vi "Set Retardation in Wave Units.vi"(0 "VISA resource name":refnum<visa-resource-name>="COM1", 1 "fraction of wave":dbl min=0.0 max=1.0 step=0.001, 3 "error in (no error)":errorcluster) -> (7 "VISA resource name out":refnum<visa-resource-name>, 10 "error out":errorcluster)   [LabVIEW 2017]
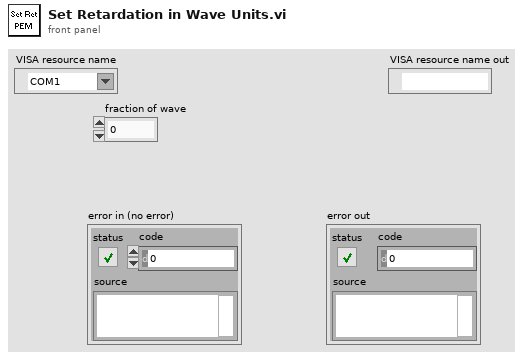
[diagram p1: front panel]
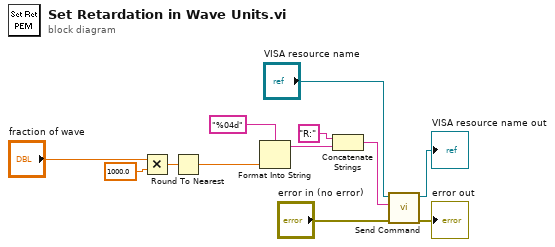
[diagram p0: block diagram]
diagram:
  n1 = Multiply(x="fraction of wave", y=1000.0) -> (x*y=w7:dbl)
  n2 = Round To Nearest(number=w7) -> (nearest integer value=w6:dbl)
  n3 = Format Into String(format string="%04d", w6) -> (resulting string=w10:string)  [unwired: 2 in, 1 out]
  n4 = Concatenate Strings("R:" ("write buffer"), w10) -> (w4:string)
  n5 = call "Send Command.vi"("error in (no error)"="error in (no error)", "write buffer"=w4, "VISA resource name"="VISA resource name") -> ("error out"=→"error out":errorcluster, "VISA resource name out"=→"VISA resource name out":refnum<visa-resource-name>)  [unwired: 7 in]
